vi "Define_Indicies_of_Affected_Tracks-1.vi"(4 "error IN":errorcluster, 5 "[IN] Subtracks":T2(array[cluster]), 6 "[IN] Indicies of sub\ntracks for transforma\ntion (resolving)":i32[](array[numeric]), 7 "[IN] Still connected\ntracks in group":T1) -> (0 "error OUT":errorcluster, 2 "[OUT] Indicies for Tr-\nack Reconstruction":i32[](array[numeric]))   [LabVIEW 2013]
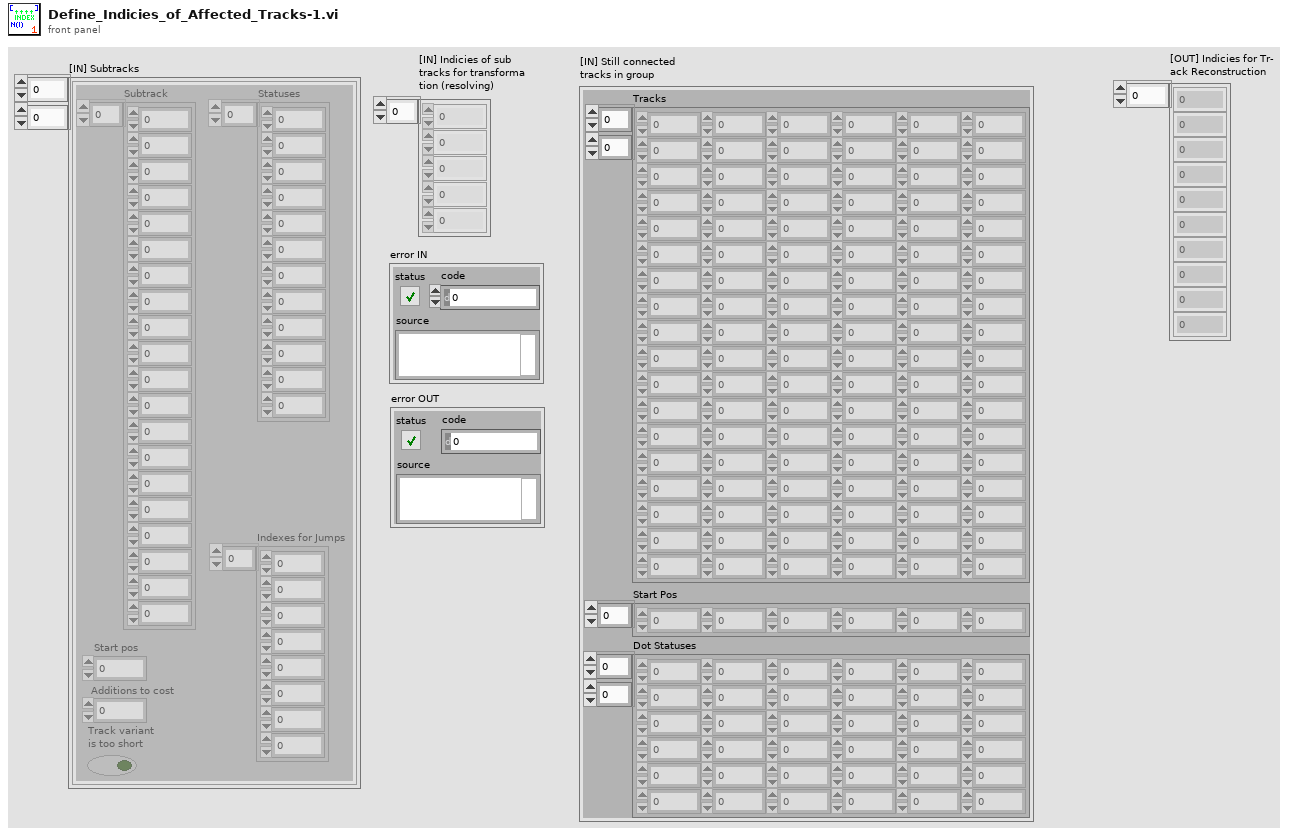
[diagram p1: front panel]
types:
  T1 = cluster{"Tracks":dbl[][], "Start Pos":i32[], "Dot Statuses":i16[][]}
  T2 = cluster{"Subtrack":dbl[], "Statuses":i16[], "Start pos":i32, "Additions to cost":i32, "Track variant \nis too short":bool, "Indexes for Jumps":i32[]}[][]
  T3 = cluster{"Subtrack":dbl[], "Statuses":i16[], "Start pos":i32, "Additions to cost":i32, "Track variant \nis too short":bool, "Indexes for Jumps":i32[]}
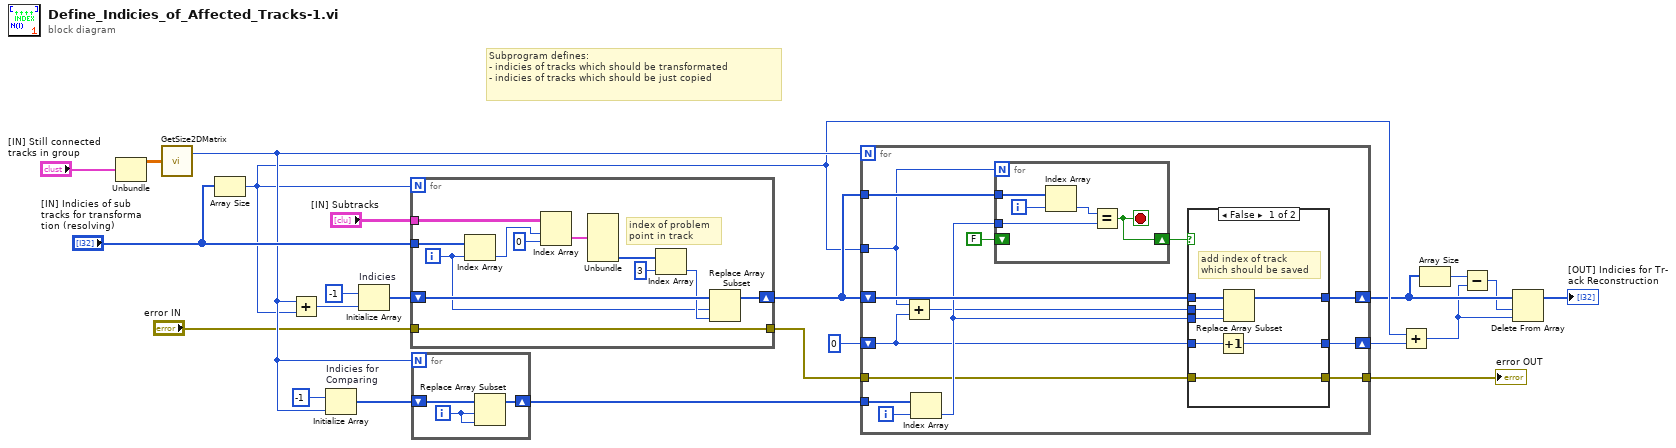
[diagram p0: block diagram]
diagram:
  # "Subprogram defines:\n- indicies of tracks which should be transformated\n- indicies of tracks which should be just copied"
  n1 = Unbundle("[IN] Still connected\ntracks in group") -> ("Tracks"=w20:dbl[][])  [unwired: 2 out]
  n2 = call "GetSize2DMatrix.vi"("Array IN (2D)"=w20) -> ("# Cols"=w13:i32)  [unwired: 1 out]
  n3 = Array Size(array="[IN] Indicies of sub\ntracks for transforma\ntion (resolving)") -> (size(s)=w10:i32)
  n4 = Add(x=w13, y=w10) -> (x+y=w19:i32)
  n5 = Initialize Array "Indicies for \nComparing"(-1 ("# Cols"), w13) -> (w15:i32[])
  n6 = Initialize Array "Indicies"(-1 ("# Cols"), w19) -> (w17:i32[])
  n7 = for {
    N: w10 -> [_]
    tunnel: "[IN] Subtracks" -> [w34]
    tunnel: "[IN] Indicies of sub\ntracks for transforma\ntion (resolving)" -> [w33]
    shift-right: [w25] -> w12
    shift-left: w17 -> [w28]
    tunnel: "error IN" -> [w24]
    tunnel: [w24] -> w2
    i -> [w26]
    # "index of problem \npoint in track"
    n8 = Index Array(array=w33, index=w26) -> (element=w32:i32)
    n9 = Index Array(array=w34, index (row)=w32, index (col)=0 ("disabled index (col)")) -> (element=w31:T3)
    n10 = Unbundle(w31) -> ("Indexes for Jumps"=w30:i32[])  [unwired: 5 out]
    n11 = Index Array(array=w30, index=3) -> (element=w27:i32)
    n12 = Replace Array Subset(array=w28, new element=w27, index=w26) -> (w25:i32[])
  }
  n13 = for {
    N: w13 -> [_]
    shift-right: [w36] -> w14
    shift-left: w15 -> [w38]
    i -> [w37]
    n14 = Replace Array Subset(array=w38, new element=w37, index=w37) -> (w36:i32[])
  }
  n15 = for {
    N: w13 -> [_]
    tunnel: w10 -> [w44]
    shift-right: [w46] -> w8
    shift-left: w12 -> [w47]
    tunnel: w14 -> [w52]
    tunnel: w12 -> [w50]
    shift-right: [w41] -> w9
    shift-left: 0 -> [w42]
    tunnel: w2 -> [w40]
    tunnel: [w39] -> w1
    i -> [w51]
    n16 = Add(x=w44, y=w42) -> (x+y=w43:i32)
    n17 = Index Array(array=w52, index=w51) -> (element=w45:i32)
    n18 = for {
      N: w44 -> [_]
      tunnel: w50 -> [w67]
      tunnel: w45 -> [w64]
      shift-right: [w63] -> w48
      shift-left: FALSE -> [_]
      i -> [w66]
      stop <- w63 stop-if-true
      n19 = Index Array(array=w67, index=w66) -> (element=w65:i32)
      n20 = Equal?(x=w65, y=w64) -> (x = y?=w63:bool)
    }
    n21 = case shown="False" w48 {
      tunnel: w47 -> [w59 w62]
      tunnel: [w56 w62] -> w46
      tunnel: w45 -> [w58 _]
      tunnel: w43 -> [w57 _]
      tunnel: w42 -> [w55 w61]
      tunnel: [w54 w61] -> w41
      tunnel: w40 -> [w53 w60]
      tunnel: [w53 w60] -> w39
      frame False {
        # "add index of track\nwhich should be saved"
        n22 = Increment(x=w55) -> (x+1=w54:i32)
        n23 = Replace Array Subset(array=w59, new element=w58, index=w57) -> (w56:i32[])
      }
      frame True {
      }
    }
  }
  "error OUT" <- w1
  n24 = Add(x=w10, y=w9) -> (x+y=w6:i32)
  n25 = Array Size(array=w8) -> (size(s)=w7:i32)
  n26 = Subtract(x=w7, y=w6) -> (x-y=w5:i32)
  n27 = Delete From Array(array=w8, length=w5, index=w6) -> (array with subset deleted=→"[OUT] Indicies for Tr-\nack Reconstruction":i32[])  [unwired: 1 out]
